vi "gauss.vi"() -> ()   [LabVIEW 2016]
uses:
  <vilib>/Analysis/2dsp.llb/2D Real FFT.vi
  <vilib>/Analysis/2dsp.llb/2D Inverse Real FFT.vi
  Gauss.dll
  <vilib>/Analysis/NI_AALPro.lvlib
panel:
  out "Array 3":dbl[][](array[numeric])
  in  "Array 2":dbl[](array[numeric])
  out "g":dbl[](array[numeric])
  in  "Show picture":u16(ring) items=["Input", "Output"]
  out "?":T1(plugin-control)
  in  "Iteratons number":dbl
  in  "sigma":dbl=50.0
  in  "kernel":i32=3
  in  "Select mode":u16(ring) items=["Standard LabView Constructions", "DLL", "Sub-device", "Standard LabView Constructions", ""]
  in  "File Path":path=path "C:/Users/Public/Pictures/Sample Pictures/Tulips.jpg"
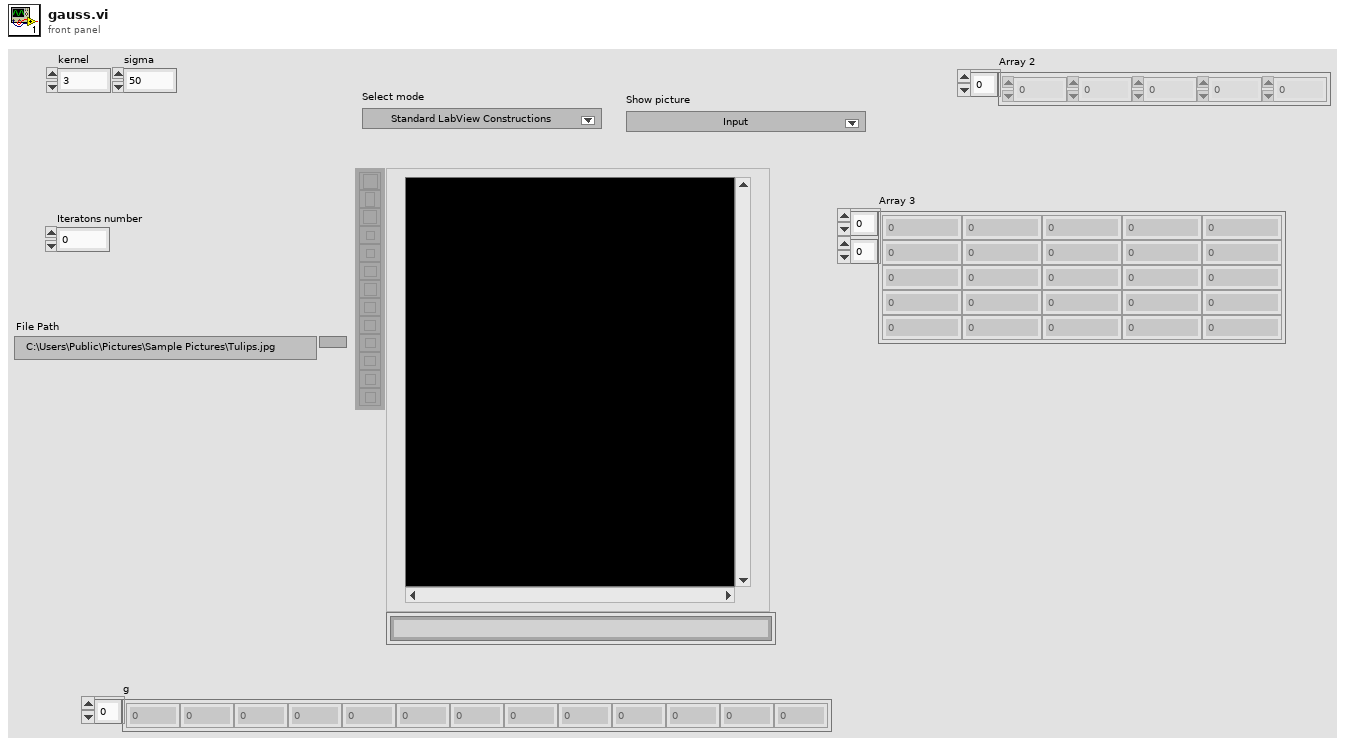
[diagram p1: front panel]
types:
  T1 = typedef "IMAQ Image.ctl" = refnum<image>
  T2 = typedef "Image Type" = u32
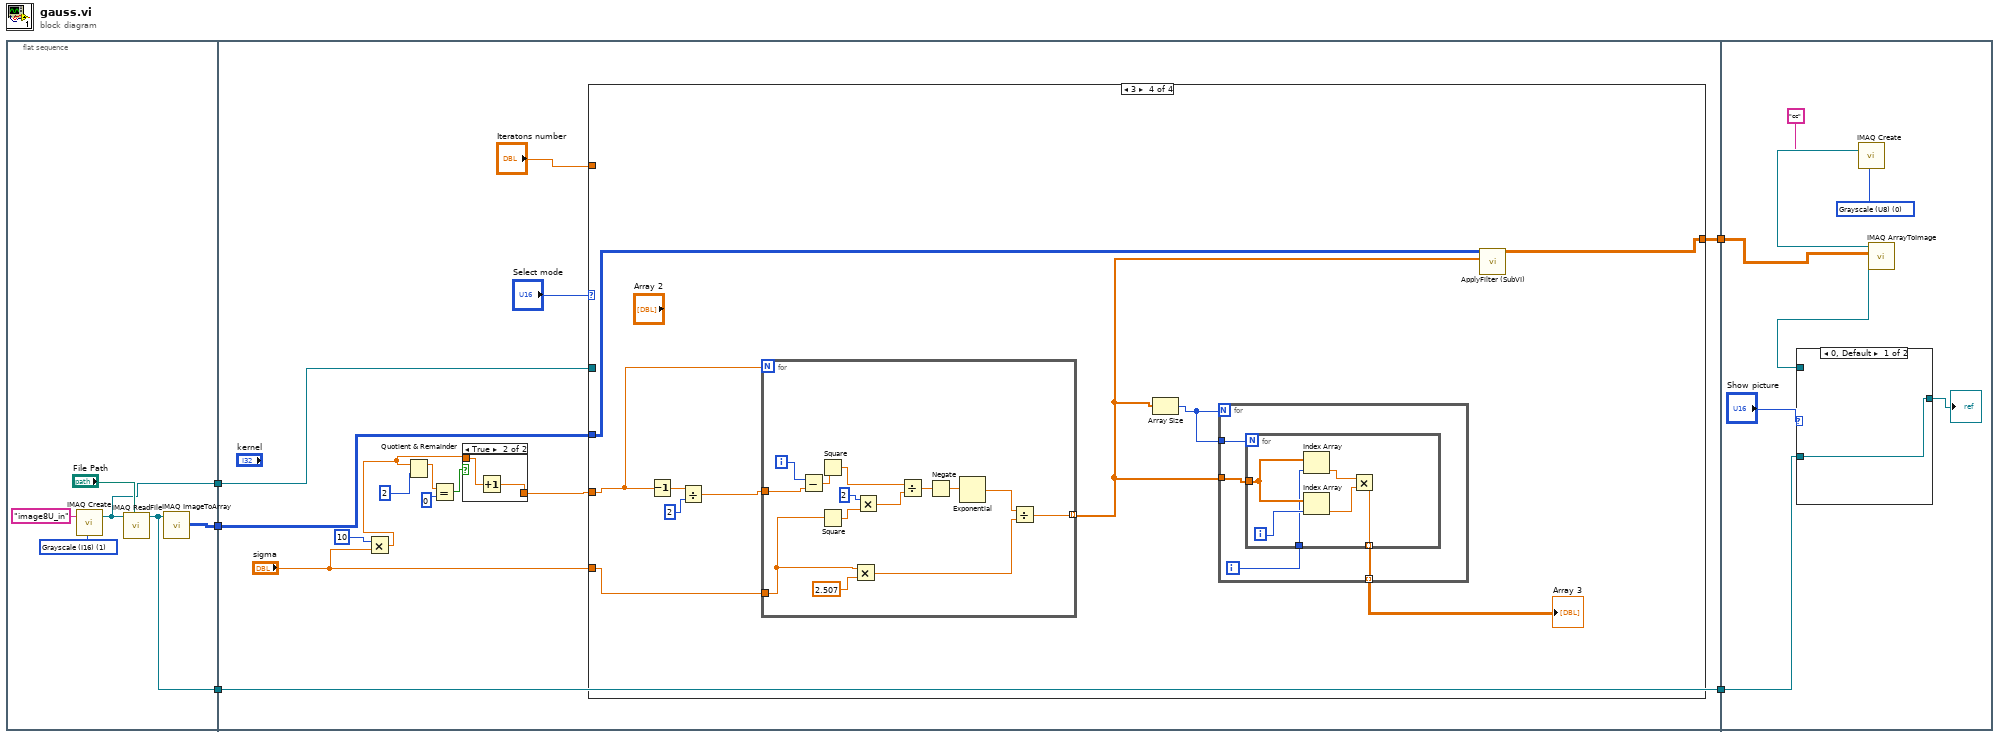
[diagram p0: block diagram]
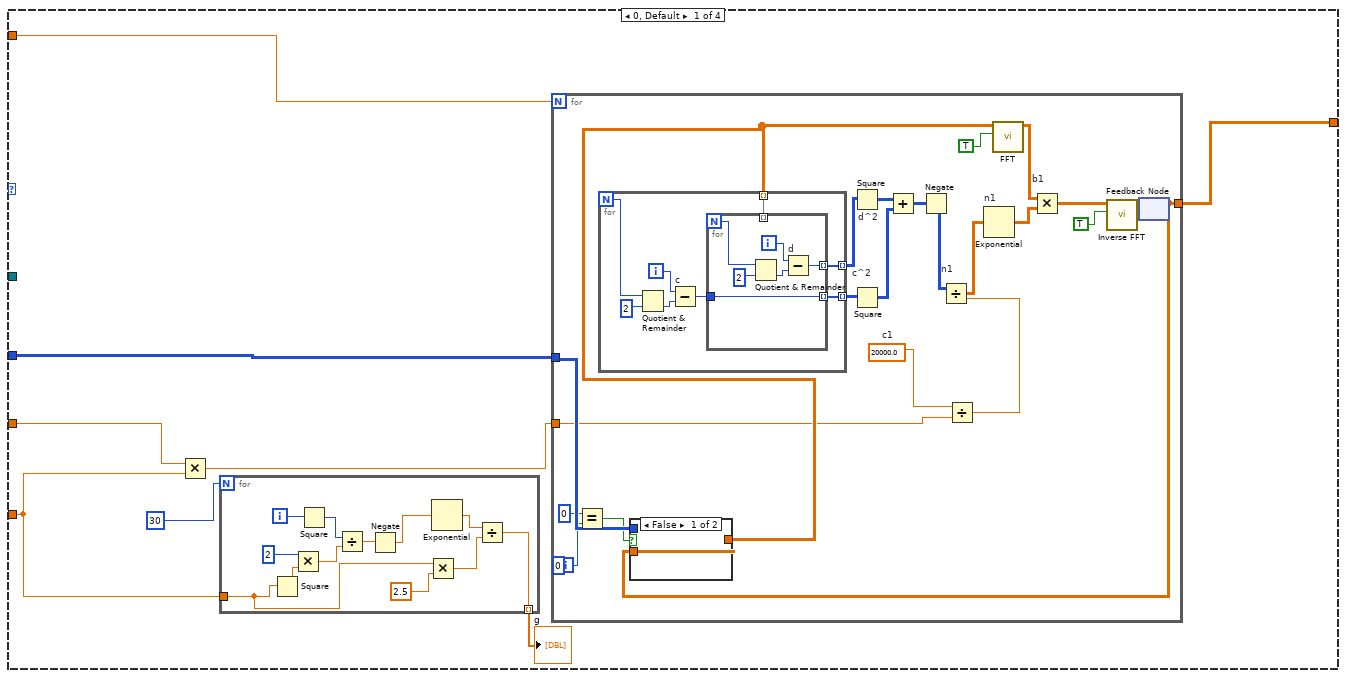
[diagram p3: hidden frame]
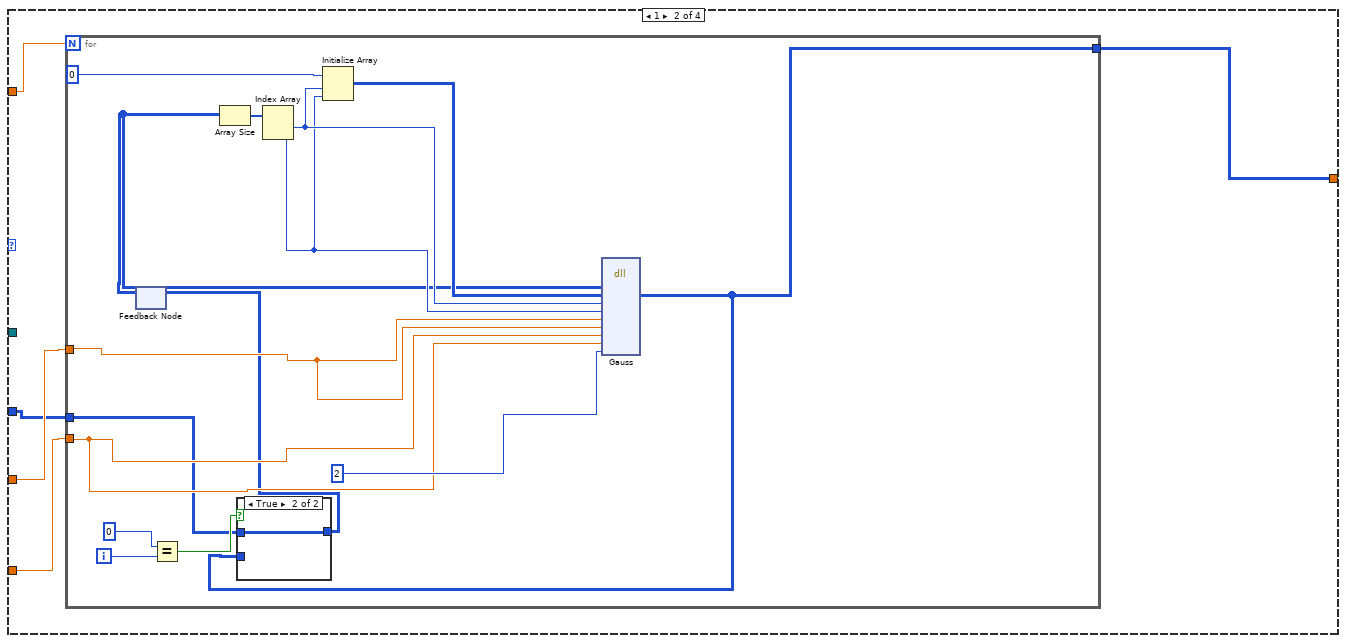
[diagram p5: hidden frame]
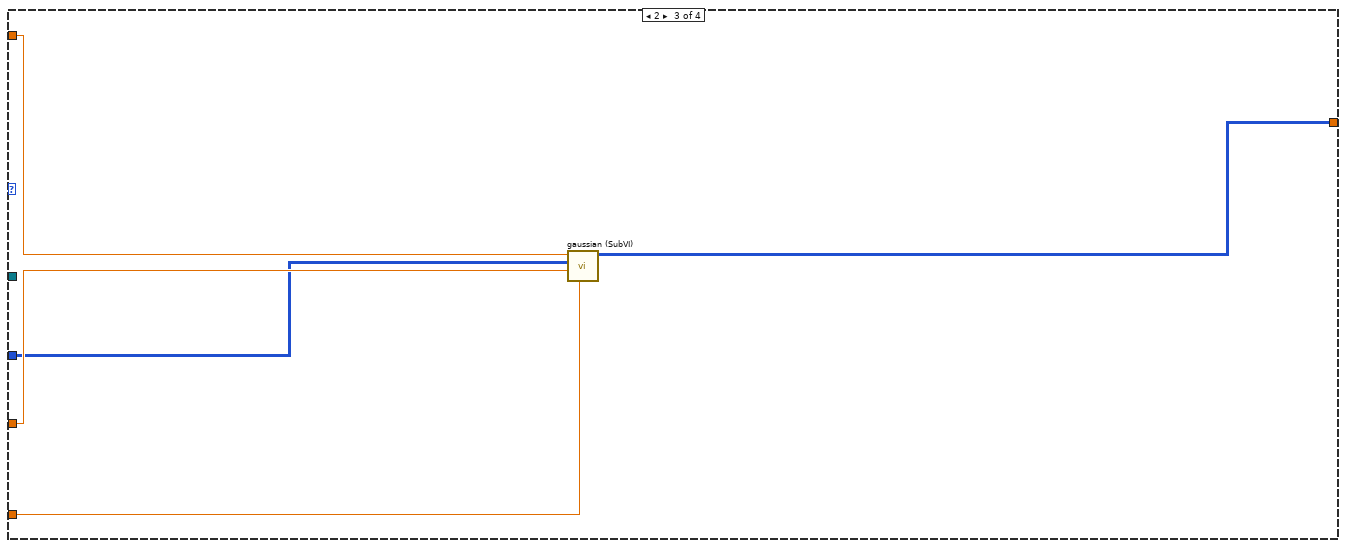
[diagram p7: hidden frame]
diagram:
  n1 = flat-sequence {
    tunnel: [w8] -> w5
    tunnel: [w7] -> w3
    tunnel: [w6] -> w1
    tunnel: w5 -> [w24]
    tunnel: [w22] -> w4
    tunnel: w3 -> [w21]
    tunnel: [w21] -> w2
    tunnel: w1 -> [w20]
    tunnel: w4 -> [w152]
    tunnel: w2 -> [w148]
    frame #0 {
      w9 = T2 1 items=["Grayscale (U8)", "Grayscale (I16)", "Grayscale (SGL)", "Complex (CSG)", "RGB (U32)", "HSL (U32)", "RGB (U64)", "Grayscale (U16)"] ("Image Type")
      n2 = call "IMAQ Create"("Image Name"="image8U_in", "Image Type"=w9) -> ("New Image"=w6:T1)  [unwired: 3 in, 1 out]
      n3 = call "IMAQ ReadFile"("File Path"="File Path", "Image"=w6) -> ("Image Out"=w7:T1)  [unwired: 5 in, 4 out]
      n4 = call "IMAQ ImageToArray"("Image"=w7) -> ("Image Pixels (I16)"=w8:i16[][])  [unwired: 3 in, 4 out]
    }
    frame #1 {
      n5 = Multiply(x=10, y="sigma") -> (x*y=w12:dbl)
      n6 = Quotient & Remainder(x=w12, y=2) -> (x-y*floor(x/y)=w18:dbl)  [unwired: 1 out]
      n7 = Equal?(x=w18, y=0) -> (x = y?=w16:bool)
      n8 = case shown="True" w16 {
        tunnel: w12 -> [w26 w28]
        tunnel: [w26 w27] -> w15
        frame False {
        }
        frame True {
          n9 = Increment(x=w28) -> (x+1=w27:dbl)
        }
      }
      n10 = case shown="3" "Select mode" {
        tunnel: w24 -> [w36 w87 w109 w123]
        tunnel: w15 -> [w33 w90 w112 w117]
        tunnel: "sigma" -> [w31 w89 w111 w121]
        tunnel: "Iteratons number" -> [w35 w88 w110 _]
        tunnel: [w34 w91 w113 w122] -> w22
        tunnel: w20 -> [_ _ _ _]
        frame 0, Default {
          n11 = Multiply(x=w33, y=w31) -> (x*y=w32:dbl)
          n12 = for {
            N: 30 -> [_]
            tunnel: w31 -> [w41]
            tunnel: [w37] -> w30 mode=indexing
            i -> [w48]
            n13 = Square(x=w41) -> (x^2=w46:dbl)
            n14 = Multiply(x=2, y=w46) -> (x*y=w45:dbl)
            n15 = Square(x=w48) -> (x^2=w44:i32)
            n16 = Divide(x=w44, y=w45) -> (x/y=w43:dbl)
            n17 = Negate(x=w43) -> (-x=w42:dbl)
            n18 = Multiply(x=w41, y=2.5) -> (x*y=w38:dbl)
            n19 = Exponential(1:w42) -> (0:w39:dbl)
            n20 = Divide(x=w39, y=w38) -> (x/y=w37:dbl)
          }
          "g" <- w30
          n21 = for {
            N: w35 -> [_]
            tunnel: w36 -> [w59]
            tunnel: [w53] -> w34
            tunnel: w32 -> [w52]
            i -> [w56]
            (unwired) 0
            w51 = 20000.0  # c1
            n22 = Equal?(x=0, y=w56) -> (x = y?=w57:bool)
            n23 = Divide(x=w51, y=w52) -> (x/y=w50:dbl)
            n24 = feedback #1() -> (w53:dbl[][])  [unwired: 1 in]
            n25 = case shown="False" w57 {
              tunnel: w59 -> [_ w72]
              tunnel: [w71 w72] -> w58
              tunnel: w53 -> [w71 _]
              frame False {
              }
              frame True {
              }
            }
            n26 = for {
              N -> [w74]
              tunnel: [w77] -> w60 mode=indexing
              tunnel: [w75] -> w61 mode=indexing
              tunnel: w58 -> [w73] mode=indexing
              i -> [w80]
              n27 = Quotient & Remainder(x=w74, y=2) -> (floor(x/y)=w78:i32)  [unwired: 1 out]
              n28 = Subtract "c"(x=w80, y=w78) -> (x-y=w76:i32)
              n29 = for {
                N -> [w81]
                tunnel: [w83] -> w77 mode=indexing
                tunnel: [w82] -> w75 mode=indexing
                tunnel: w76 -> [w82]
                tunnel: w73 -> [_] mode=indexing
                i -> [w84]
                n30 = Quotient & Remainder(x=w81, y=2) -> (floor(x/y)=w85:i32)  [unwired: 1 out]
                n31 = Subtract "d"(x=w84, y=w85) -> (x-y=w83:i32)
              }
            }
            n32 = Square "d^2"(x=w60) -> (x^2=w62:i32[][])
            n33 = Square "c^2"(x=w61) -> (x^2=w63:i32[][])
            n34 = Add(x=w62, y=w63) -> (x+y=w64:i32[][])
            n35 = Negate(x=w64) -> (-x=w66:i32[][])
            n36 = Divide "n1"(x=w66, y=w50) -> (x/y=w65:dbl[][])
            n37 = Exponential "n1"(1:w65) -> (0:w49:dbl[][])
            n38 = call-poly <vilib>:"FFT.vi"("shift?"=TRUE, "X"=w58) -> ("FFT {X}"=w70:cdb[][])  [unwired: 8 in, 1 out]
            n39 = Multiply "b1"(x=w70, y=w49) -> (x*y=w67:cdb[][])
            n40 = call-poly <vilib>:"Inverse FFT.vi"("shift?"=TRUE, "FFT {X}"=w67) -> ("X"=w54:dbl[][])  [unwired: 8 in, 1 out]
            n41 = feedback-in #1(w54) -> ()
          }
        }
        frame 1 {
          n42 = for {
            N: w88 -> [_]
            tunnel: [w94] -> w91
            tunnel: w90 -> [w100]
            tunnel: w89 -> [w99]
            tunnel: w87 -> [w95]
            i -> [w98]
            n43 = feedback #2() -> (w92:u16[][])  [unwired: 1 in]
            n44 = Equal?(x=0, y=w98) -> (x = y?=w96:bool)
            n45 = Array Size(array=w92) -> (size(s)=w103:i32[])
            n46 = Index Array(array=w103) -> (element #1=w102:i32, element #2=w101:i32)  [unwired: 2 in]
            n47 = Initialize Array(u8 0 ("element"), w102, w101) -> (w105:u8[][])
            n48 = dll-call lib="G:/bsuir/mag/prytkov/GaussianImageProcessor/Gauss.dll" fn="Gauss"("imageIN"=w92, "imageOUT"=w105, "rows"=w102, "cols"=w101, "kernelX"=w100, "kernelY"=w100, "sigmaX"=w99, "sigmaY"=w99, "borderType"=2) -> ("imageOUT"=w94:u16[][])  [unwired: 12 in, 2 out]
            n49 = case shown="True" w96 {
              tunnel: [w107 w108] -> w93
              tunnel: w95 -> [_ w108]
              tunnel: w94 -> [w107 _]
              frame False {
              }
              frame True {
              }
            }
            n50 = feedback-in #2(w93) -> ()
          }
        }
        frame 2 {
          n51 = call "gaussian (SubVI).vi"("sigma"=w111, "kernel"=w112, "Image Pixels (I16)"=w109, "Iteratons number"=w110) -> ("imageOUT"=w113:u16[][])  [unwired: 7 in]
        }
        frame 3 {
          n52 = Decrement(x=w117) -> (x-1=w119:dbl)
          n53 = Divide(x=w119, y=2) -> (x/y=w118:dbl)
          n54 = for {
            N: w117 -> [_]
            tunnel: w121 -> [w140]
            tunnel: [w137] -> w115 mode=indexing
            tunnel: w118 -> [w135]
            i -> [w136]
            n55 = Subtract(x=w136, y=w135) -> (x-y=w134:dbl)
            n56 = Square(x=w134) -> (x^2=w145:dbl)
            n57 = Square(x=w140) -> (x^2=w147:dbl)
            n58 = Multiply(x=w140, y=2.507) -> (x*y=w139:dbl)
            n59 = Multiply(x=2, y=w147) -> (x*y=w144:dbl)
            n60 = Divide(x=w145, y=w144) -> (x/y=w143:dbl)
            n61 = Negate(x=w143) -> (-x=w142:dbl)
            n62 = Exponential(1:w142) -> (0:w138:dbl)
            n63 = Divide(x=w138, y=w139) -> (x/y=w137:dbl)
          }
          n64 = Array Size(array=w115) -> (size(s)=w114:i32)
          n65 = for {
            N: w114 -> [_]
            tunnel: w115 -> [w127]
            tunnel: [w125] -> w116 mode=indexing
            tunnel: w114 -> [w124]
            i -> [w126]
            n66 = for {
              N: w124 -> [_]
              tunnel: w127 -> [w133]
              tunnel: w126 -> [w131]
              tunnel: [w128] -> w125 mode=indexing
              i -> [w132]
              n67 = Index Array(array=w133, index=w131) -> (element=w130:dbl)
              n68 = Index Array(array=w133, index=w132) -> (element=w129:dbl)
              n69 = Multiply(x=w130, y=w129) -> (x*y=w128:dbl)
            }
          }
          "Array 3" <- w116
          n70 = call "ApplyFilter (SubVI).vi"("Array in"=w115, "Image Pixels (I16)"=w123) -> ("Array out"=w122:dbl[][])  [unwired: 9 in]
        }
      }
    }
    frame #2 {
      w153 = T2 0 items=["Grayscale (U8)", "Grayscale (I16)", "Grayscale (SGL)", "Complex (CSG)", "RGB (U32)", "HSL (U32)", "RGB (U64)", "Grayscale (U16)"] ("Image Type")
      n71 = call "IMAQ Create"("Image Name"="cc", "Image Type"=w153) -> ("New Image"=w155:T1)  [unwired: 3 in, 1 out]
      n72 = call "IMAQ ArrayToImage"("Image Pixels (U8)"=w152, "Image"=w155) -> ("Image Out"=w149:T1)  [unwired: 8 in, 1 out]
      n73 = case shown="0, Default" "Show picture" {
        tunnel: [w156 w157] -> w150
        tunnel: w149 -> [_ w157]
        tunnel: w148 -> [w156 _]
        frame 0, Default {
        }
        frame 1 {
        }
      }
      "?" <- w150
    }
  }
